vi "Camera startup.vi"() -> ()   [LabVIEW 2011]
doc: "Cools down the camera to operating temperature before use and returns it to ambient after use. Run this VI before running any other ixon programs and leave it running the whole time you use the camera. To start: run vi, set temperature, check \"cooling\". To finish: Click \"warm up CCD and turn off camera\". Leave running until the program tells you that it has turned off the camera."
uses:
  ixon camera/HAL camera properties.ctl
  ixon camera/HAL cooling status.ctt
  camera globals.vi
panel:
  out "Cooling status":T1
  in  "Warm up CCD & Turn Off Camera":bool
  in  "Cooling":bool
  out "Detector Temperature":i32(graph)
  in  "Temp. Set Point":i32(slide)=-80 scale=-120.0..20.0
  out "Camera Properties":T2
  out "Status":string
  in  "error in (no error)":errorcluster
  # "Camera:  Andor iXon"
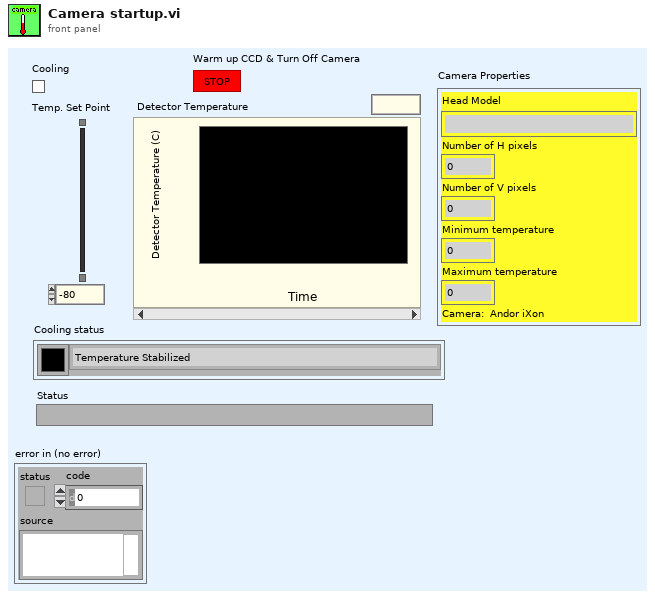
[diagram p1: front panel]
types:
  T1 = typedef "HAL cooling status.ctt" = cluster{"Color Box":u32, "Cooling Status":enum16{"Temperature Stabilized", "Waiting to Stabilize Temperature", "Cooling is Turned Off", "Have not yet Reached Set Temperature"}}
  T2 = typedef "HAL camera properties.ctl" = cluster{"Head Model":string, "Number of H pixels":i32, "Number of V pixels":i32, "Minimum temperature":i32, "Maximum temperature":i32}
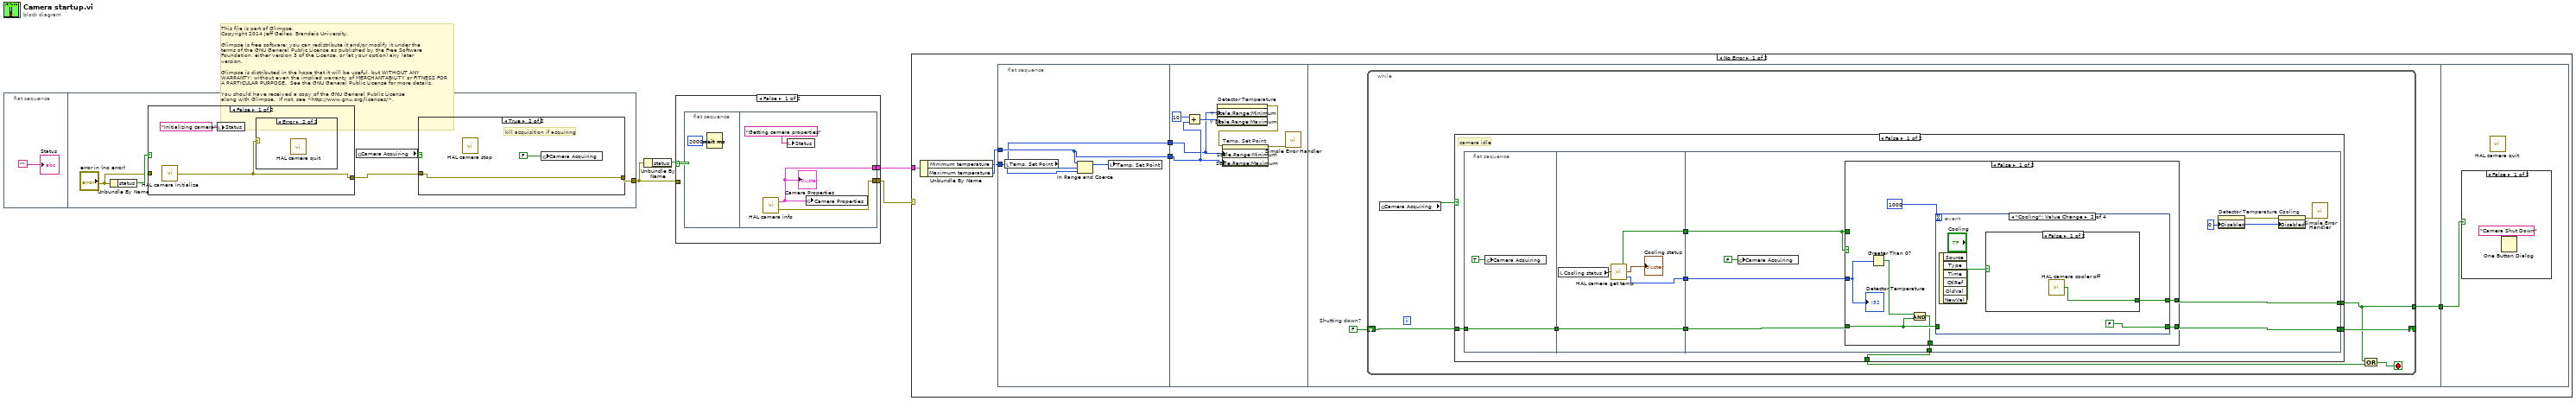
[diagram p0: block diagram]
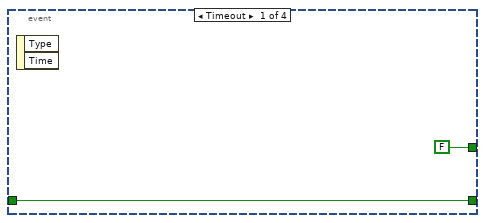
[diagram p2: hidden frame]
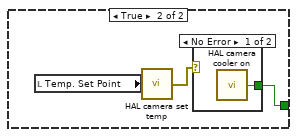
[diagram p3: hidden frame]
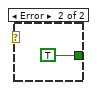
[diagram p4: hidden frame]
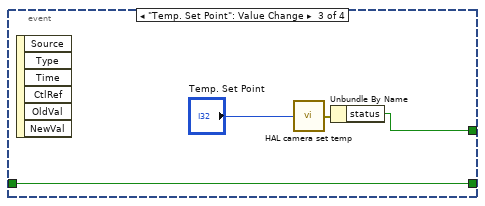
[diagram p5: hidden frame]
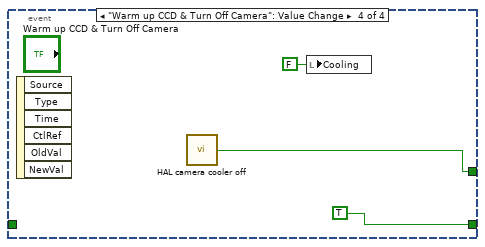
[diagram p6: hidden frame]
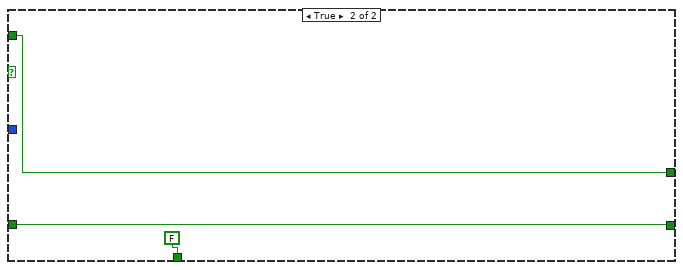
[diagram p7: hidden frame]
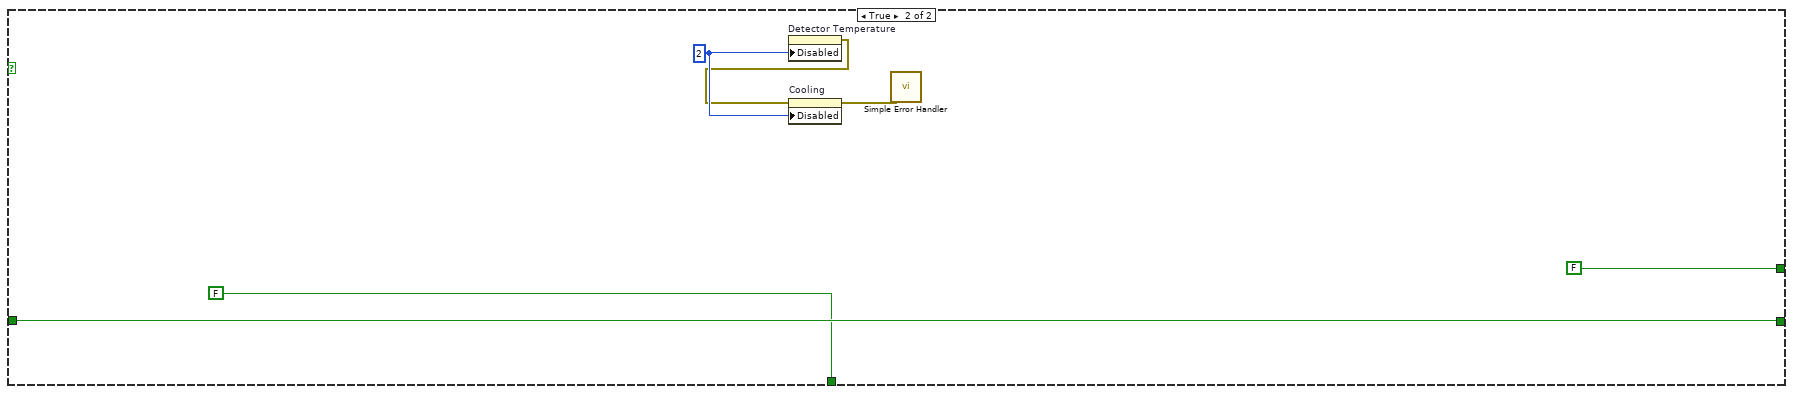
[diagram p8: hidden frame]
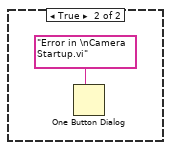
[diagram p9: hidden frame]
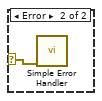
[diagram p10: hidden frame]
diagram:
  # "This file is part of Glimpse. \nCopyright 2014 Jeff Gelles, Brandeis University.    \n\nGlimpse is free software: you can redistribute it and/or modify it under the \nterms of the GNU General Public License as published by the Free Software \nFoundation, either version 3 of the License, or (at your option) any later \nversion.\n\nGlimpse is distributed in the hope that it will be useful, but WITHOUT ANY \nWARRANTY; without even the implied warranty of MERCHANTABILITY or FITNESS FOR \nA PARTICULAR PURPOSE.  See the GNU General Public License for more details.\n\nYou should have received a copy of the GNU General Public License\nalong with Glimpse.  If not, see <http://www.gnu.org/licenses/>."
  n1 = flat-sequence {
    tunnel: [w7] -> w3
    frame #0 {
      "Status" <- ""
    }
    frame #1 {
      n2 = Unbundle By Name("error in (no error)") -> ("status"=w10:bool)
      n3 = case shown="False" w10 {
        tunnel: [w14 w16] -> w8
        tunnel: "error in (no error)" -> [_ w16]
        frame False {
          n4 = call "HAL camera initialize.vi"() -> ("error out"=w14:errorcluster)
          n5 = local write "Status"("Initializing camera" ("Status")) -> ()
          n6 = case shown="Error" w14 {
            frame No Error {
            }
            frame Error {
              n7 = call "HAL camera quit.vi"() -> ()  [unwired: 1 out]
            }
          }
        }
        frame True {
        }
      }
      n8 = global read "camera globals.vi" "Camera Acquiring"() -> (w6:bool)
      n9 = case shown="True" w6 {
        tunnel: [w11 w13] -> w7
        tunnel: w8 -> [w11 w13]
        frame False {
        }
        frame True {
          # "kill acquisition if acquiring"
          n10 = call "HAL camera stop.vi"() -> ()  [unwired: 1 out]
          n11 = global write "camera globals.vi" "Camera Acquiring"(FALSE ("Andor Aquiring")) -> ()
        }
      }
    }
  }
  n12 = Unbundle By Name(w3) -> ("status"=w4:bool)
  n13 = case shown="False" w4 {
    tunnel: [w17 w23] -> w1
    tunnel: w3 -> [_ w23]
    tunnel: [w18 _] -> w2
    frame False {
      n14 = flat-sequence {
        tunnel: [w20] -> w18
        tunnel: [w21] -> w17
        frame #0 {
          n15 = Wait (ms)(milliseconds to wait=u32 2000) -> ()  [unwired: 1 out]
        }
        frame #1 {
          n16 = call "HAL camera info.vi"() -> ("error out"=w21:errorcluster, "Andor Camera Properties"=w20:T2)  [unwired: 2 in]
          "Camera Properties" <- w20
          n17 = local write "Status"("Getting camera properties" ("Status")) -> ()
          n18 = global write "camera globals.vi" "Camera Properties"(w20) -> ()
        }
      }
    }
    frame True {
    }
  }
  n19 = case shown="No Error" w1 {
    selector: w1 -> [_ w110]
    tunnel: w2 -> [w29 _]
    frame No Error {
      n20 = Unbundle By Name(w29) -> ("Minimum temperature"=w25:i32, "Maximum temperature"=w27:i32)
      n21 = flat-sequence {
        tunnel: w27 -> [w31]
        tunnel: [w31] -> w26
        tunnel: w25 -> [w30]
        tunnel: [w30] -> w24
        tunnel: w26 -> [w35]
        tunnel: w24 -> [w34]
        tunnel: [w40] -> w28
        tunnel: w28 -> [w107]
        frame #0 {
          n22 = local read "Temp. Set Point"() -> (w33:i32)
          n23 = In Range and Coerce(upper limit=w31, x=w33, lower limit=w30) -> (coerced(x)=w32:i32)  [unwired: 1 out]
          n24 = local write "Temp. Set Point"(w32) -> ()
        }
        frame #1 {
          n25 = Add(x=10, y=w35) -> (x+y=w38:i32)
          n26 = property on="Detector Temperature" class="WFChart (strict)"("Y Scale.Range:Minimum"=w34, "Y Scale.Range:Maximum"=w38) -> (error out=w37:errorcluster)  [unwired: 2 in, 1 out]
          n27 = property on="Temp. Set Point" class="Slide (strict)"(error in=w37, "Scale.Range:Minimum"=w34, "Scale.Range:Maximum"=w35) -> (error out=w36:errorcluster)  [unwired: 1 in, 1 out]
          n28 = call <vilib>:"Simple Error Handler.vi"("error in (no error)"=w36) -> ()  [unwired: 1 in, 8 out]
        }
        frame #2 {
          w41 = FALSE  # Shutting down?
          n29 = while {
            shift-right: [w45] -> _
            shift-left: w41 -> [w46]
            tunnel: [w42] -> w40
            stop <- w43 stop-if-true
            n30 = global read "camera globals.vi" "Camera Acquiring"() -> (w47:bool)
            n31 = case shown="False" w47 {
              tunnel: w46 -> [w52 w104]
              tunnel: [w55 w104] -> w45
              tunnel: [w54 FALSE] -> w44
              tunnel: [w53 FALSE ("status")] -> w42
              frame False {
                # "camera idle"
                n32 = flat-sequence {
                  tunnel: w52 -> [w57]
                  tunnel: [w57] -> w51
                  tunnel: w51 -> [w62]
                  tunnel: [w62] -> w50
                  tunnel: [w59] -> w49
                  tunnel: [w58] -> w48
                  tunnel: [w69] -> w55
                  tunnel: [w68] -> w54
                  tunnel: [w67] -> w53
                  tunnel: w50 -> [w66]
                  tunnel: w49 -> [w65]
                  tunnel: w48 -> [w64]
                  frame #0 {
                    n33 = global write "camera globals.vi" "Camera Acquiring"(TRUE ("Camera Acquiring")) -> ()
                  }
                  frame #1 {
                    n34 = local read "Cooling status"() -> (w61:T1)
                    n35 = call "HAL camera get temp.vi"("Cooling status In"=w61) -> ("Error?"=w59:bool, "Cooling status Out"=→"Cooling status":T1, "Current temperature"=w58:i32)
                  }
                  frame #2 {
                    w72 = u8 0 ("Disabled")
                    n36 = global write "camera globals.vi" "Camera Acquiring"(FALSE ("Camera Acquiring")) -> ()
                    n37 = case shown="False" w65 {
                      tunnel: [w78 w98] -> w69
                      tunnel: w66 -> [w77 w98]
                      tunnel: w64 -> [w76 _]
                      tunnel: [w74 FALSE] -> w68
                      tunnel: [w73 w100] -> w67
                      tunnel: w65 -> [_ w100]
                      frame False {
                        n38 = Greater Than 0?(x=w76) -> (x > 0?=w75:bool)
                        n39 = And(x=w75, y=w77) -> (x .and. y?=w74:bool)
                        n40 = event shown="[1] \"Cooling\": Value Change" {
                          selector: _ -> [_ _ _ _]
                          dyn-events: _ -> [_ _ _ _]
                          timeout: 1000 -> [_ _ _ _]
                          tunnel: w77 -> [w81 _ w91 _]
                          tunnel: [w81 FALSE w91 TRUE] -> w78
                          tunnel: [FALSE ("status") w83 w92 w96] -> w73
                          event Timeout {
                            n41 = event-data() -> ()  [unwired: 3 out]
                          }
                          event "Cooling": Value Change {
                            n42 = event-data() -> ("NewVal"=w82:bool)  [unwired: 6 out]
                            n43 = case shown="False" w82 {
                              tunnel: [w85 w88] -> w83
                              frame False {
                                n44 = call "HAL camera cooler off.vi"() -> ("Error?"=w85:bool)
                              }
                              frame True {
                                n45 = local read "Temp. Set Point"() -> (w87:i32)
                                n46 = call "HAL camera set temp.vi"("Temp. Set Point"=w87) -> ("error out"=w86:errorcluster)
                                n47 = case shown="No Error" w86 {
                                tunnel: [w89 TRUE ("error?")] -> w88
                                frame No Error {
                                n48 = call "HAL camera cooler on.vi"() -> ("error?"=w89:bool)
                                }
                                frame Error {
                                }
                                }
                              }
                            }
                          }
                          event "Temp. Set Point": Value Change {
                            n49 = event-data() -> ()  [unwired: 7 out]
                            n50 = call "HAL camera set temp.vi"("Temp. Set Point"="Temp. Set Point") -> ("error out"=w93:errorcluster)
                            n51 = Unbundle By Name(w93) -> ("status"=w92:bool)
                          }
                          event "Warm up CCD & Turn Off Camera": Value Change {
                            n52 = event-data() -> ()  [unwired: 7 out]
                            n53 = call "HAL camera cooler off.vi"() -> ("Error?"=w96:bool)
                            n54 = local write "Cooling"(FALSE ("Cooling")) -> ()
                          }
                        }
                        "Detector Temperature" <- w76
                      }
                      frame True {
                      }
                    }
                    n55 = property on="Detector Temperature" class="WFChart (strict)"("Disabled"=w72) -> (error out=w71:errorcluster)  [unwired: 2 in, 1 out]
                    n56 = property on="Cooling" class="Bool (strict)"(error in=w71, "Disabled"=w72) -> (error out=w70:errorcluster)  [unwired: 1 in, 1 out]
                    n57 = call <vilib>:"Simple Error Handler.vi"("error in (no error)"=w70) -> ()  [unwired: 1 in, 8 out]
                  }
                }
              }
              frame True {
                w106 = u8 2 ("Disabled")
                n58 = property on="Detector Temperature" class="WFChart (strict)"("Disabled"=w106) -> (error out=w105:errorcluster)  [unwired: 2 in, 1 out]
                n59 = property on="Cooling" class="Bool (strict)"(error in=w105, "Disabled"=w106) -> (error out=w101:errorcluster)  [unwired: 1 in, 1 out]
                n60 = call <vilib>:"Simple Error Handler.vi"("error in (no error)"=w101) -> ()  [unwired: 1 in, 8 out]
              }
            }
            n61 = Compound Arithmetic op=OR(w42, w44) -> (w43:bool)
          }
        }
        frame #3 {
          n62 = case shown="False" w107 {
            frame False {
              n63 = One Button Dialog(message="Camera Shut Down" ("string")) -> ()  [unwired: 2 out]
            }
            frame True {
              n64 = One Button Dialog(message="Error in \nCamera Startup.vi" ("string")) -> ()  [unwired: 2 out]
            }
          }
          n65 = call "HAL camera quit.vi"() -> ()  [unwired: 1 out]
        }
      }
    }
    frame Error {
      n66 = call <vilib>:"Simple Error Handler.vi"("error in (no error)"=w110) -> ()  [unwired: 1 in, 8 out]
    }
  }
